vi "FormatDataForReport.vi"(6 "Report selection":i32, 8 "error in (no error)":errorcluster, 10 "Path":path) -> (0 "error out":errorcluster, 1 "Data":dbl[][](array[numeric]), 2 "Names":string[](array[string]), 3 "Activity armpressure":dbl[](array[numeric]), 4 "output cluster":cluster{"Names":string[], "Data":dbl[][]}, 5 "Normal armpressure":dbl[](array[numeric]))   [LabVIEW 2013, in "main.lvlib"]
uses:
  main.lvlib
  <vilib>/Analysis/baseanly.llb/Mean (DBL).vi
  <vilib>/Analysis/NI_AALBase.lvlib
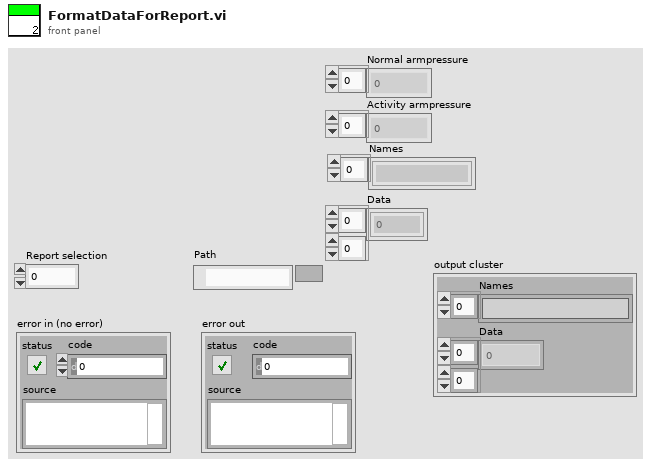
[diagram p1: front panel]
types:
  T1 = cluster{"sys":dbl, "dia":dbl, "puls":dbl, "date":string, "time":string, "code":string, "serial":string, "temp":dbl, "activity":string}[]
  T2 = cluster{"Non-activity":cluster{"Sys":dbl[], "Dia":dbl[], "Puls":dbl[], "Temp":dbl[], "Date":string[], "Time":string[]}, "Activity":cluster{"Sys":dbl[], "Dia":dbl[], "Puls":dbl[], "Temp":dbl[], "Date":string[], "Time":string[]}}
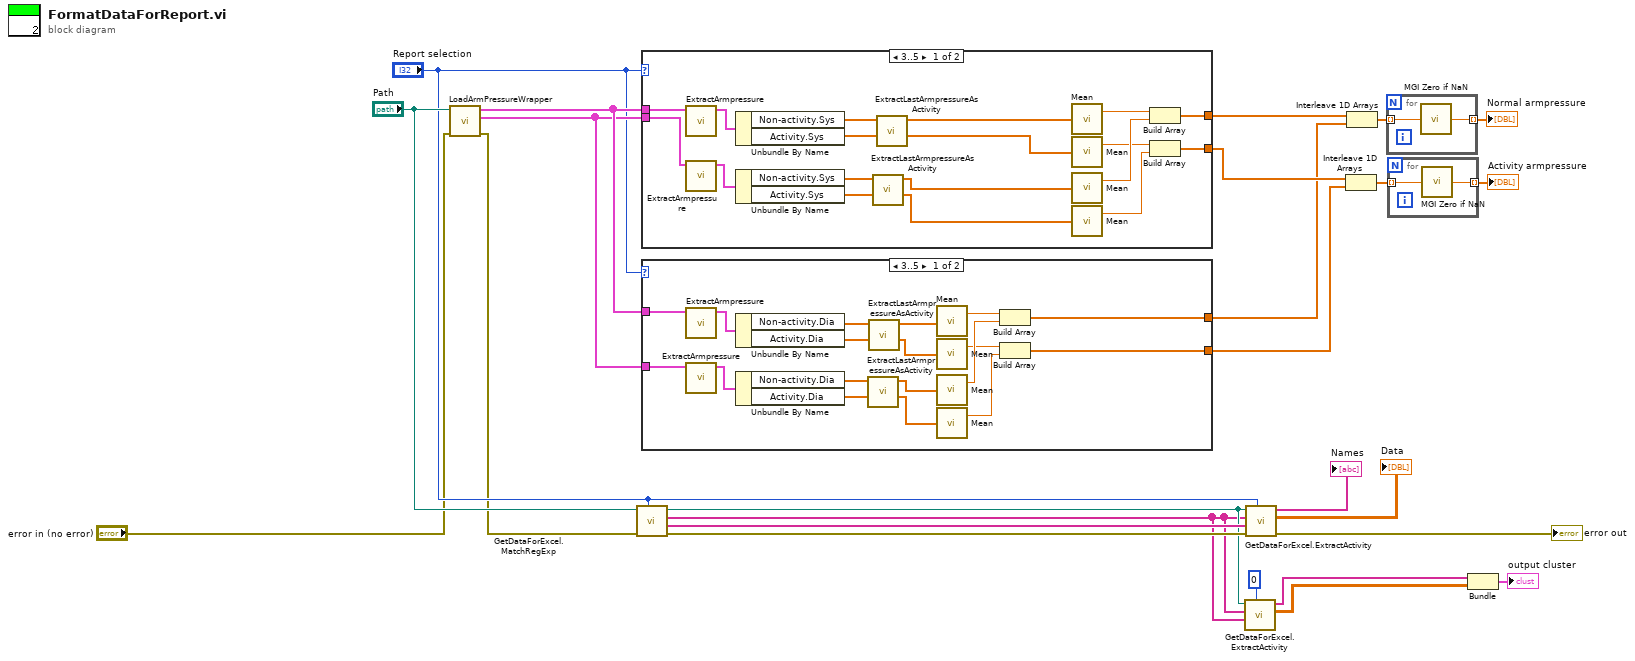
[diagram p0: block diagram]
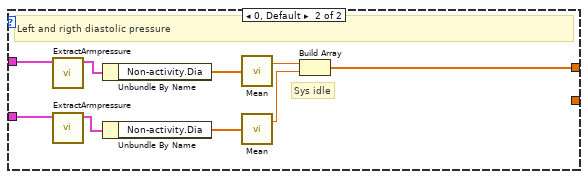
[diagram p2: hidden frame]
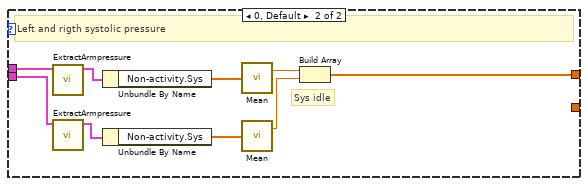
[diagram p3: hidden frame]
diagram:
  n1 = call "LoadArmPressureWrapper.vi"("error in"="error in (no error)", "File dir"="Path") -> ("error out"=w14:errorcluster, "Armpressure Left"=w21:T1, "Armpressure Right"=w22:T1)  [unwired: 7 in]
  n2 = call "GetDataForExcel.MatchRegExp.vi"("Journal"="Report selection", "error in"=w14, "path"="Path") -> ("error out"=w25:errorcluster, "Active"=w24:string[], "Normal"=w5:string[], "path out"=w6:path)  [unwired: 5 in]
  n3 = case shown="3..5" "Report selection" {
    tunnel: w22 -> [w43 w52]
    tunnel: w21 -> [w42 w51]
    tunnel: [w36 w44] -> w17
    tunnel: [w35 _] -> w20
    frame 3..5 {
      n4 = call "ExtractArmpressure.vi"("Arm pressure"=w43) -> ("output cluster"=w40:T2)  [unwired: 10 in]
      n5 = call "ExtractArmpressure.vi"("Arm pressure"=w42) -> ("output cluster"=w41:T2)  [unwired: 10 in]
      n6 = Unbundle By Name(w40) -> ("Non-activity.Sys"=w34:dbl[], "Activity.Sys"=w32:dbl[])
      n7 = Unbundle By Name(w41) -> ("Non-activity.Sys"=w30:dbl[], "Activity.Sys"=w29:dbl[])
      n8 = call "ExtractLastArmpressureAsActivity.vi"("Activity"=w29, "Non-activity"=w30) -> ("Activity"=w27:dbl[], "Non-activity"=w28:dbl[])  [unwired: 8 in]
      n9 = call "ExtractLastArmpressureAsActivity.vi"("Activity"=w32, "Non-activity"=w34) -> ("Activity"=w31:dbl[], "Non-activity"=w33:dbl[])  [unwired: 8 in]
      n10 = call-poly <vilib>:"Mean.vi"("X"=w33) -> ("mean"=w26:dbl)  [unwired: 1 out]
      n11 = call-poly <vilib>:"Mean.vi"("X"=w31) -> ("mean"=w38:dbl)  [unwired: 1 out]
      n12 = call-poly <vilib>:"Mean.vi"("X"=w28) -> ("mean"=w39:dbl)  [unwired: 1 out]
      n13 = call-poly <vilib>:"Mean.vi"("X"=w27) -> ("mean"=w37:dbl)  [unwired: 1 out]
      n14 = Build Array(w26, w39) -> (w36:dbl[])
      n15 = Build Array(w38, w37) -> (w35:dbl[])
    }
    frame 0, Default {
      # "Sys idle"
      # "Left and rigth systolic pressure"
      n16 = call "ExtractArmpressure.vi"("Arm pressure"=w52) -> ("output cluster"=w49:T2)  [unwired: 10 in]
      n17 = call "ExtractArmpressure.vi"("Arm pressure"=w51) -> ("output cluster"=w50:T2)  [unwired: 10 in]
      n18 = Unbundle By Name(w49) -> ("Non-activity.Sys"=w48:dbl[])
      n19 = Unbundle By Name(w50) -> ("Non-activity.Sys"=w47:dbl[])
      n20 = call-poly <vilib>:"Mean.vi"("X"=w48) -> ("mean"=w46:dbl)  [unwired: 1 out]
      n21 = call-poly <vilib>:"Mean.vi"("X"=w47) -> ("mean"=w45:dbl)  [unwired: 1 out]
      n22 = Build Array(w46, w45) -> (w44:dbl[])
    }
  }
  n23 = case shown="3..5" "Report selection" {
    tunnel: [w64 w73] -> w16
    tunnel: [w63 _] -> w19
    tunnel: w22 -> [w62 w72]
    tunnel: w21 -> [w61 w71]
    frame 3..5 {
      n24 = call "ExtractArmpressure.vi"("Arm pressure"=w62) -> ("output cluster"=w69:T2)  [unwired: 10 in]
      n25 = call "ExtractArmpressure.vi"("Arm pressure"=w61) -> ("output cluster"=w70:T2)  [unwired: 10 in]
      n26 = Unbundle By Name(w69) -> ("Non-activity.Dia"=w60:dbl[], "Activity.Dia"=w59:dbl[])
      n27 = Unbundle By Name(w70) -> ("Non-activity.Dia"=w58:dbl[], "Activity.Dia"=w57:dbl[])
      n28 = call "ExtractLastArmpressureAsActivity.vi"("Activity"=w57, "Non-activity"=w58) -> ("Activity"=w53:dbl[], "Non-activity"=w54:dbl[])  [unwired: 8 in]
      n29 = call "ExtractLastArmpressureAsActivity.vi"("Activity"=w59, "Non-activity"=w60) -> ("Activity"=w55:dbl[], "Non-activity"=w56:dbl[])  [unwired: 8 in]
      n30 = call-poly <vilib>:"Mean.vi"("X"=w56) -> ("mean"=w68:dbl)  [unwired: 1 out]
      n31 = call-poly <vilib>:"Mean.vi"("X"=w55) -> ("mean"=w66:dbl)  [unwired: 1 out]
      n32 = call-poly <vilib>:"Mean.vi"("X"=w54) -> ("mean"=w67:dbl)  [unwired: 1 out]
      n33 = call-poly <vilib>:"Mean.vi"("X"=w53) -> ("mean"=w65:dbl)  [unwired: 1 out]
      n34 = Build Array(w68, w67) -> (w64:dbl[])
      n35 = Build Array(w66, w65) -> (w63:dbl[])
    }
    frame 0, Default {
      # "Sys idle"
      # "Left and rigth diastolic pressure"
      n36 = call "ExtractArmpressure.vi"("Arm pressure"=w72) -> ("output cluster"=w78:T2)  [unwired: 10 in]
      n37 = call "ExtractArmpressure.vi"("Arm pressure"=w71) -> ("output cluster"=w79:T2)  [unwired: 10 in]
      n38 = Unbundle By Name(w78) -> ("Non-activity.Dia"=w77:dbl[])
      n39 = Unbundle By Name(w79) -> ("Non-activity.Dia"=w76:dbl[])
      n40 = call-poly <vilib>:"Mean.vi"("X"=w77) -> ("mean"=w75:dbl)  [unwired: 1 out]
      n41 = call-poly <vilib>:"Mean.vi"("X"=w76) -> ("mean"=w74:dbl)  [unwired: 1 out]
      n42 = Build Array(w75, w74) -> (w73:dbl[])
    }
  }
  n43 = call "GetDataForExcel.ExtractActivity.vi"("ReportSelection"=u16 0, "Active"=w5, "Normal"=w5, "path in"=w6) -> ("Data"=w2:dbl[][], "Names"=w3:string[])  [unwired: 5 in, 1 out]
  n44 = call "GetDataForExcel.ExtractActivity.vi"("ReportSelection"="Report selection", "error in (no error)"=w25, "Active"=w24, "Normal"=w5, "path in"=w6) -> ("error out"=→"error out":errorcluster, "Data"=→"Data":dbl[][], "Names"=→"Names":string[])  [unwired: 4 in]
  n45 = Interleave 1D Arrays(w20, w19) -> (w12:dbl[])
  n46 = Interleave 1D Arrays(w17, w16) -> (w13:dbl[])
  n47 = for {
    tunnel: w13 -> [w81] mode=indexing
    tunnel: [w80] -> w10 mode=indexing
    n48 = call <userlib>:"MGI Zero if NaN.vi"("Number In"=w81) -> ("Number Out"=w80:dbl)
  }
  "Normal armpressure" <- w10
  n49 = for {
    tunnel: w12 -> [w83] mode=indexing
    tunnel: [w82] -> w9 mode=indexing
    n50 = call <userlib>:"MGI Zero if NaN.vi"("Number In"=w83) -> ("Number Out"=w82:dbl)
  }
  "Activity armpressure" <- w9
  n51 = Bundle("Names"=w3, "Data"=w2) -> (→"output cluster":cluster{"Names":string[], "Data":dbl[][]})  [unwired: 1 in]
